vi "ExportPacketToJSON.vi"(6 "DefaultFolderName(Data)":string="Data", 7 "Prompt":string caption="prompt", 8 "Comment":string, 9 "NumerOfSamplesForAxis":i32, 10 "GyroData":waveform(dbl)[](array[waveform]), 11 "AccelData":waveform(dbl)[](array[waveform])) -> (0 "ErrorOut":errorcluster, 1 "Exported?":bool)   [LabVIEW 2016]
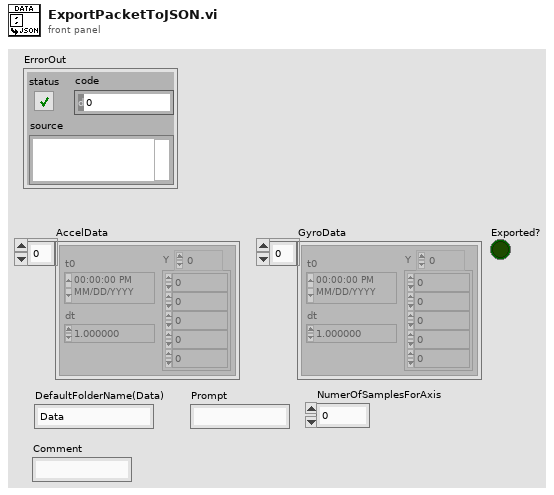
[diagram p1: front panel]
types:
  T1 = enum16{"open", "replace", "create", "open or create", "replace or create", "replace or create with confirmation"}
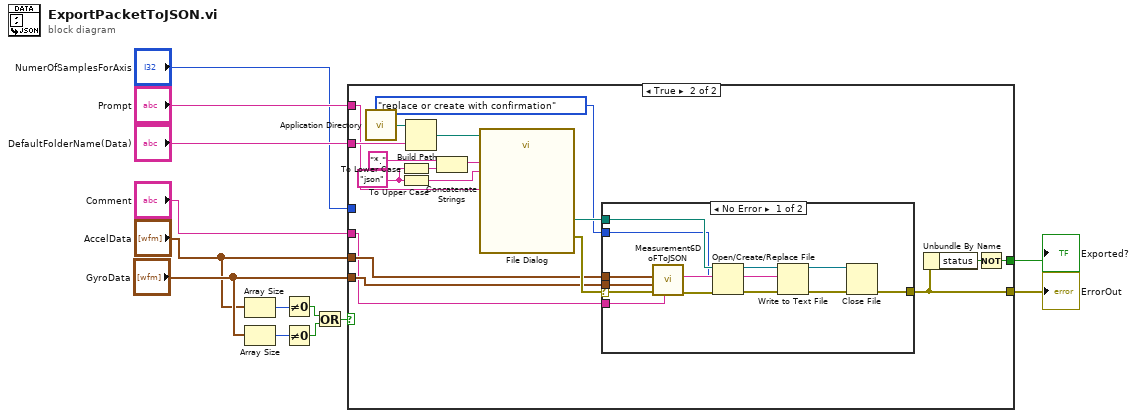
[diagram p0: block diagram]
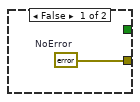
[diagram p2: hidden frame]
diagram:
  n1 = Array Size(array="AccelData") -> (size(s)=w8:i32)
  n2 = Array Size(array="GyroData") -> (size(s)=w9:i32)
  n3 = Not Equal To 0?(x=w8) -> (x != 0?=w6:bool)
  n4 = Not Equal To 0?(x=w9) -> (x != 0?=w5:bool)
  n5 = Or(x=w6, y=w5) -> (x .or. y?=w4:bool)
  n6 = case shown="True" w4 {
    tunnel: "DefaultFolderName(Data)" -> [_ w32]
    tunnel: [w14 w18] -> w12
    tunnel: "Prompt" -> [_ w23]
    tunnel: "GyroData" -> [_ w19]
    tunnel: "AccelData" -> [_ w20]
    tunnel: "NumerOfSamplesForAxis" -> [_ _]
    tunnel: [_ w16] -> w2
    tunnel: "Comment" -> [_ w15]
    frame False {
      w14 = errorcluster {"status"=FALSE, "code"=0, "source"=""}  # NoError
    }
    frame True {
      w25 = "json" ("string")
      n7 = call <vilib>:"Application Directory.vi"() -> ("Application Directory"=w31:path)
      n8 = To Lower Case(string=w25) -> (all lower case string=w28:string)
      n9 = To Upper Case(1:w25) -> (0:w29:string)
      n10 = Build Path(base path=w31, name or relative path=w32) -> (appended path=w30:path)
      n11 = Concatenate Strings("*." ("string"), w28) -> (w26:string)
      n12 = call "File Dialog"("start path"=w30, "prompt"=w23, "pattern (all files)"=w26, "pattern label"=w29) -> ("selected path"=w24:path, "error out"=w21:errorcluster)  [unwired: 8 in, 2 out]
      n13 = case shown="No Error" w21 {
        selector: w21 -> [w39 w46]
        tunnel: [w45 w46] -> w18
        tunnel: w24 -> [w44 _]
        tunnel: T1."replace or create with confirmation" ("operation (0:open)") -> [w34 _]
        tunnel: w20 -> [w38 _]
        tunnel: w19 -> [w37 _]
        tunnel: w15 -> [w33 _]
        frame No Error {
          n14 = call "Measurement6DoFToJSON.vi"("Comment"=w33, "ErrorIn"=w39, "GyroData"=w37, "AccelData"=w38) -> ("ErrorOut"=w36:errorcluster, "JSONMeasurement6DoF"=w35:string)  [unwired: 5 in, 1 out]
          n15 = Open/Create/Replace File(file path (use dialog)=w44, error in=w36, operation (0:open)=w34) -> (refnum out=w42:refnum<file>, error out=w43:errorcluster)  [unwired: 3 in, 1 out]
          n16 = Write to Text File(file (use dialog)=w42, text=w35, error in=w43) -> (refnum out=w40:refnum<file>, error out=w41:errorcluster)  [unwired: 1 in, 1 out]
          n17 = Close File(refnum=w40, error in=w41) -> (error out=w45:errorcluster)  [unwired: 1 out]
        }
        frame Error {
        }
      }
      n18 = Unbundle By Name(w18) -> ("status"=w17:bool)
      n19 = Not(x=w17) -> (.not. x?=w16:bool)
    }
  }
  "ErrorOut" <- w12
  "Exported?" <- w2
